vi "Save_reference_Raw_data.vi"(6 "Data_struct":refnum<k24>[](array[refnum]), 7 "chkeach_ch":bool, 8 "错误输入（无错误）":errorcluster, 9 "Ref_monitordata_struct":refnum<k24>[](array[refnum]), 10 "Refdata_struct":refnum<k24>[](array[refnum]), 11 "PDLSTS":refnum<k24>) -> (0 "错误输出":errorcluster)   [LabVIEW 2017]
doc: "Save reference Raw data"
uses:
  D:/test/PDLSTS/LV_PDL_Sample/DLL/STSProcess.dll
  DLL/STSProcess.dll
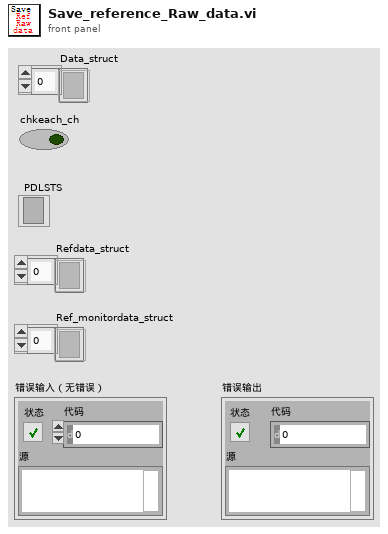
[diagram p1: front panel]
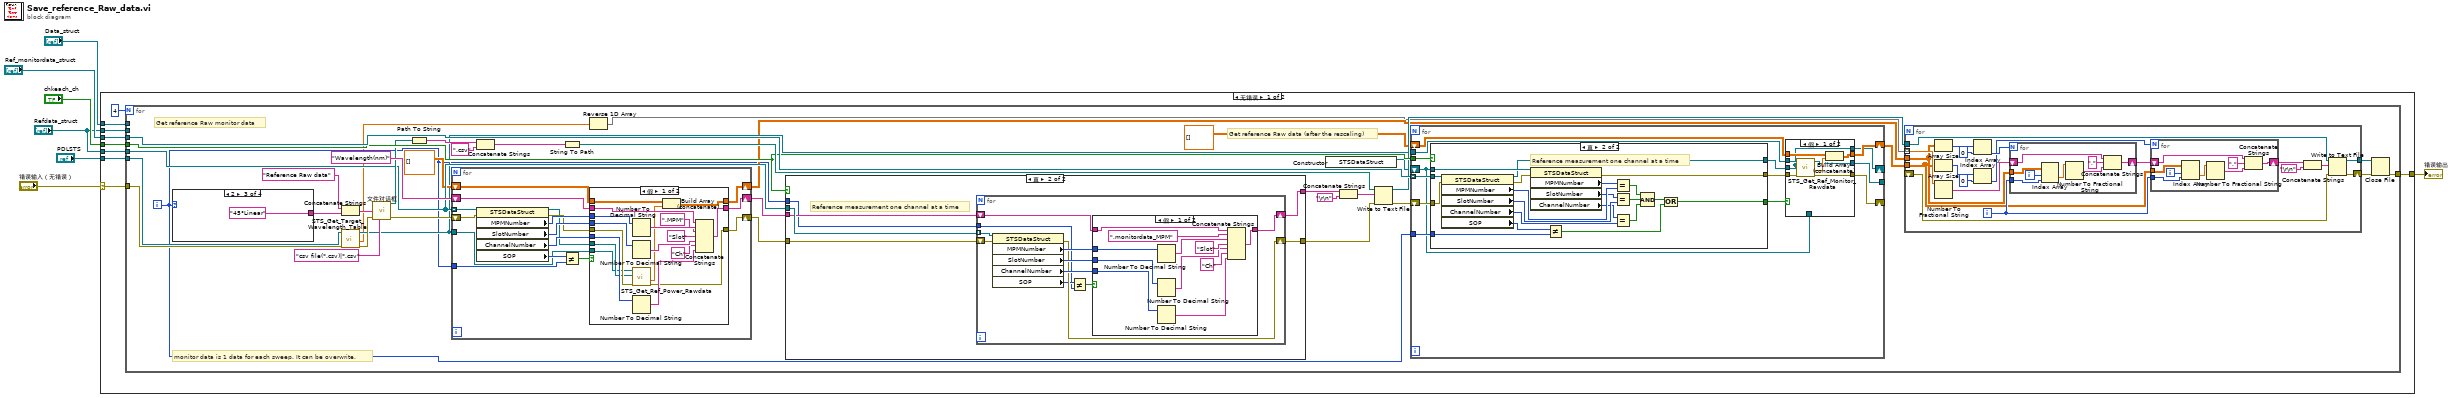
[diagram p0: block diagram]
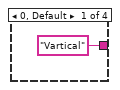
[diagram p2: hidden frame]
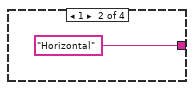
[diagram p3: hidden frame]
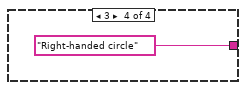
[diagram p4: hidden frame]
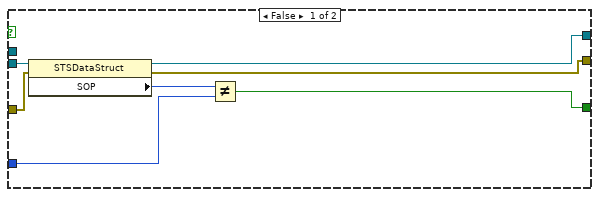
[diagram p6: hidden frame]
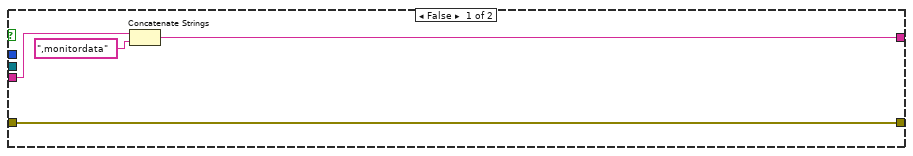
[diagram p7: hidden frame]
diagram:
  n1 = case shown="无错误" "错误输入（无错误）" {
    selector: "错误输入（无错误）" -> [w10 w216]
    tunnel: [w11 w216] -> w7
    tunnel: "Ref_monitordata_struct" -> [w16 _]
    tunnel: "chkeach_ch" -> [w13 _]
    tunnel: "PDLSTS" -> [w9 _]
    tunnel: "Refdata_struct" -> [w15 _]
    tunnel: "Data_struct" -> [w14 _]
    tunnel: "Refdata_struct" -> [w12 _]
    frame No Error {
      n2 = for {
        N: 4 -> [_]
        tunnel: w16 -> [w53]
        tunnel: w15 -> [_]
        tunnel: w14 -> [_]
        tunnel: w13 -> [w44]
        tunnel: w12 -> [w24]
        tunnel: [w36] -> w11
        tunnel: w10 -> [w32]
        tunnel: w9 -> [w31]
        i -> [w19]
        # "Get reference Raw monitor data"
        # "monitor data is 1 data for each sweep. It can be overwrite."
        # "Get reference Raw data (after the rescaling)"
        n3 = case shown="2" w19 {
          tunnel: ["Vartical" "Horizontal" "45°Linear" "Right-handed circle"] -> w27
          frame 0, Default {
          }
          frame 1 {
          }
          frame 2 {
          }
          frame 3 {
          }
        }
        n4 = Concatenate Strings("Reference Raw data" ("字符串"), w27) -> (w26:string)
        n5 = call "STS_Get_Target_Wavelength_Table.vi"("错误输入（无错误）"=w32, ".NET引用句柄输入"=w31) -> ("error out"=w25:errorcluster, "wavelengths"=w18:dbl[], "引用输出"=w22:refnum<k24>)  [unwired: 7 in]
        n6 = call "文件对话框"("default name"=w26, "error in"=w25, "pattern (all files)"="csv file(*.csv)|*.csv") -> ("selected path"=w30:path, "error out"=w48:errorcluster)  [unwired: 9 in, 2 out]
        n7 = Path To String(path=w30) -> (string=w29:string)
        n8 = for {
          tunnel: w24 -> [w194] mode=indexing
          shift-right: [w188] -> w43
          shift-left: "Wavelength(nm)" -> [w189]
          shift-right: [w181] -> w42
          shift-left: w48 -> [w193]
          tunnel: w19 -> [w185]
          shift-right: [w183] -> w20
          shift-left: sgl[][] [] -> [w184]
          tunnel: w22 -> [w179]
          n9 = property on="属性节点" class="STSDataStruct"(reference=w194, error in=w193) -> (reference out=w180:refnum<k24>, error out=w182:errorcluster, "MPMNumber"=w190:i32, "SlotNumber"=w191:i32, "ChannelNumber"=w192:i32, "SOP"=w187:i32)
          n10 = Not Equal?(x=w187, y=w185) -> (x != y?=w186:bool)
          n11 = case shown="假" w186 {
            tunnel: w192 -> [w212 _]
            tunnel: w191 -> [w211 _]
            tunnel: w190 -> [w210 _]
            tunnel: w189 -> [w209 w215]
            tunnel: [w202 w215] -> w188
            tunnel: w184 -> [w201 w214]
            tunnel: [w199 w214] -> w183
            tunnel: w182 -> [w198 w213]
            tunnel: [w197 w213] -> w181
            tunnel: w180 -> [w196 _]
            tunnel: w179 -> [w195 _]
            frame False {
              n12 = Number To Decimal String(number=w210) -> (decimal integer string=w207:string)  [unwired: 1 in]
              n13 = Number To Decimal String(number=w211) -> (decimal integer string=w205:string)  [unwired: 1 in]
              n14 = call "STS_Get_Ref_Power_Rawdata.vi"("错误输入（无错误）"=w198, "setting"=w196, ".NET引用句柄输入"=w195) -> ("error out"=w197:errorcluster, "powerdata"=w200:sgl[])  [unwired: 6 in, 1 out]
              n15 = Number To Decimal String(number=w212) -> (decimal integer string=w203:string)  [unwired: 1 in]
              n16 = Build Array (concatenate)(w201, w200) -> (w199:sgl[][])
              n17 = Concatenate Strings(w209, ",MPM" ("字符串"), w207, "Slot" ("字符串"), w205, "Ch" ("字符串"), w203) -> (w202:string)
            }
            frame True {
            }
          }
        }
        n18 = Concatenate Strings(w29, ".csv" ("名称或相对路径")) -> (w46:string)
        n19 = String To Path(string=w46) -> (path=w45:path)
        n20 = Reverse 1D Array(array=w18) -> (reversed array=w17:dbl[])
        n21 = case shown="真" w44 {
          tunnel: w24 -> [_ w154]
          tunnel: w43 -> [w149 w153]
          tunnel: w42 -> [w146 w155]
          tunnel: [w147 w152] -> w41
          tunnel: [w146 w151] -> w40
          tunnel: w19 -> [_ w150]
          frame False {
            n22 = Concatenate Strings(w149, ",monitordata" ("字符串")) -> (w147:string)
          }
          frame True {
            # "Reference measurement one channel at a time"
            n23 = for {
              tunnel: w154 -> [w166] mode=indexing
              shift-right: [w160] -> w152
              shift-left: w153 -> [w161]
              shift-right: [w159] -> w151
              shift-left: w155 -> [w165]
              tunnel: w150 -> [w157]
              n24 = property on="属性节点" class="STSDataStruct"(reference=w166, error in=w165) -> (error out=w159:errorcluster, "MPMNumber"=w162:i32, "SlotNumber"=w163:i32, "ChannelNumber"=w164:i32, "SOP"=w158:i32)  [unwired: 1 out]
              n25 = Not Equal?(x=w158, y=w157) -> (x != y?=w156:bool)
              n26 = case shown="假" w156 {
                tunnel: w164 -> [w177 _]
                tunnel: w163 -> [w176 _]
                tunnel: w162 -> [w175 _]
                tunnel: w161 -> [w174 w178]
                tunnel: [w167 w178] -> w160
                frame False {
                  n27 = Number To Decimal String(number=w175) -> (decimal integer string=w172:string)  [unwired: 1 in]
                  n28 = Number To Decimal String(number=w176) -> (decimal integer string=w170:string)  [unwired: 1 in]
                  n29 = Number To Decimal String(number=w177) -> (decimal integer string=w168:string)  [unwired: 1 in]
                  n30 = Concatenate Strings(w174, ",monitordata_MPM" ("字符串"), w172, "Slot" ("字符串"), w170, "Ch" ("字符串"), w168) -> (w167:string)
                }
                frame True {
                }
              }
            }
          }
        }
        n31 = constructor class="STSDataStruct"() -> (reference out=w33:refnum<k24>)  [unwired: 3 in, 2 out]
        n32 = Concatenate Strings(w41, "\r\n") -> (w51:string)
        n33 = Write to Text File(file (use dialog)=w45, text=w51, error in=w40) -> (refnum out=w39:refnum<file>, error out=w21:errorcluster)  [unwired: 1 in, 1 out]
        n34 = for {
          tunnel: w44 -> [w106]
          tunnel: w53 -> [w105] mode=indexing
          shift-right: [w97] -> _
          shift-left: w21 -> [w104]
          shift-right: [w94] -> _
          shift-left: w33 -> [w93]
          tunnel: w22 -> [w101]
          shift-right: [w100] -> w34
          shift-left: sgl[][] [] -> [w99]
          tunnel: [w96] -> _
          tunnel: w19 -> [w95]
          n35 = case shown="真" w106 {
            tunnel: w105 -> [w125 w145]
            tunnel: w104 -> [w124 w144]
            tunnel: w93 -> [_ w143]
            tunnel: [w119 w126] -> w103
            tunnel: [w123 w132] -> w102
            tunnel: [w122 w131] -> w98
            tunnel: w95 -> [w120 w129]
            frame False {
              n36 = property on="属性节点" class="STSDataStruct"(reference=w125, error in=w124) -> (reference out=w122:refnum<k24>, error out=w123:errorcluster, "SOP"=w121:i32)
              n37 = Not Equal?(x=w121, y=w120) -> (x != y?=w119:bool)
            }
            frame True {
              # "Reference measurement one channel at a time"
              n38 = property on="属性节点" class="STSDataStruct"(reference=w145, error in=w144) -> (reference out=w131:refnum<k24>, error out=w142:errorcluster, "MPMNumber"=w140:i32, "SlotNumber"=w138:i32, "ChannelNumber"=w137:i32, "SOP"=w130:i32)
              n39 = property class="STSDataStruct"(reference=w143, error in=w142) -> (error out=w132:errorcluster, "MPMNumber"=w141:i32, "SlotNumber"=w139:i32, "ChannelNumber"=w136:i32)  [unwired: 1 out]
              n40 = Not Equal?(x=w130, y=w129) -> (x != y?=w128:bool)
              n41 = Equal?(x=w141, y=w140) -> (x = y?=w135:bool)
              n42 = Equal?(x=w139, y=w138) -> (x = y?=w134:bool)
              n43 = Equal?(x=w136, y=w137) -> (x = y?=w133:bool)
              n44 = Compound Arithmetic op=AND ("复合运算")(w135, w134, w133) -> (w127:bool)
              n45 = Compound Arithmetic op=OR ("复合运算")(w127, w128) -> (w126:bool)
            }
          }
          n46 = case shown="假" w103 {
            tunnel: w102 -> [w114 w117]
            tunnel: w98 -> [w107 _]
            tunnel: w101 -> [w113 w116]
            tunnel: [w111 w118] -> w100
            tunnel: w99 -> [w110 w118]
            tunnel: [w109 w117] -> w97
            tunnel: [w108 w116] -> w96
            tunnel: [w107 w115] -> w94
            tunnel: w93 -> [_ w115]
            frame False {
              n47 = call "STS_Get_Ref_Monitor_Rawdata.vi"("错误输入（无错误）"=w114, "setting"=w107, ".NET引用句柄输入"=w113) -> ("error out"=w109:errorcluster, "monitordata"=w112:sgl[], "引用输出"=w108:refnum<k24>)  [unwired: 6 in]
              n48 = Build Array (concatenate)(w110, w112) -> (w111:sgl[][])
            }
            frame True {
            }
          }
        }
        n49 = for {
          tunnel: w17 -> [w76] mode=indexing
          tunnel: w34 -> [w59]
          tunnel: w39 -> [w68]
          tunnel: [w67] -> w38
          tunnel: w20 -> [w66]
          shift-right: [w73] -> w37
          shift-left: _ -> [w74]
          i -> [w62]
          n50 = Array Size(array=w66) -> (size(s)=w71:i32[])
          n51 = Array Size(array=w59) -> (size(s)=w61:i32[])
          n52 = Number To Fractional String(number=w76) -> (F-format string=w75:string)  [unwired: 3 in]
          n53 = Index Array(array=w71, index=0 ("索引")) -> (element=w69:i32)
          n54 = Index Array(array=w61, index=0 ("索引")) -> (element=w58:i32)
          n55 = for {
            N: w69 -> [_]
            tunnel: w66 -> [w92]
            tunnel: w62 -> [w91]
            shift-right: [w87] -> w64
            shift-left: w75 -> [w88]
            i -> [w90]
            n56 = Index Array(array=w92, index (row)=w90, index (col)=w91) -> (element=w89:sgl)
            n57 = Number To Fractional String(number=w89) -> (F-format string=w85:string)  [unwired: 3 in]
            n58 = Concatenate Strings(w88, "," ("字符串"), w85) -> (w87:string)
          }
          n59 = for {
            N: w58 -> [_]
            tunnel: w59 -> [w84]
            tunnel: w62 -> [w83]
            shift-right: [w79] -> w63
            shift-left: w64 -> [w80]
            i -> [w82]
            n60 = Index Array(array=w84, index (row)=w82, index (col)=w83) -> (element=w81:sgl)
            n61 = Number To Fractional String(number=w81) -> (F-format string=w77:string)  [unwired: 3 in]
            n62 = Concatenate Strings(w80, "," ("字符串"), w77) -> (w79:string)
          }
          n63 = Concatenate Strings(w63, "\r\n") -> (w72:string)
          n64 = Write to Text File(file (use dialog)=w68, text=w72, error in=w74) -> (refnum out=w67:refnum<file>, error out=w73:errorcluster)  [unwired: 1 in, 1 out]
        }
        n65 = Close File(refnum=w38, error in=w37) -> (error out=w36:errorcluster)  [unwired: 1 out]
      }
    }
    frame Error {
    }
  }
  "错误输出" <- w7
